vi "Send Cyclic to gRPC.vi"(8 "error in (no error)":errorcluster, 11 "CIFTemplatePlugin in":refnum<class "TemplatePlugin.lvclass">) -> (0 "error out":errorcluster, 3 "CIFTemplatePlugin out":refnum<class "TemplatePlugin.lvclass">)   [LabVIEW 2021, in "TemplatePlugin.lvclass"]
uses:
  TemplatePlugin.lvclass
  C:/Program Files/National Instruments/LabVIEW 2021/vi.lib/CIF Foundation/CIF Core/CIFCore/Class/CIFCorePlugin.lvclass
  <vilib>/CIF Foundation/CIF Core/CIFCore/Class/CIFCorePlugin.lvclass/CIFCorePlugin.ctl
  TemplatePlugin.lvclass/TemplatePlugin.ctl
  0c0f428d-7269-422d-ba27-f9d6fa7232ec.vi
  <vilib>/CIF Foundation/CIF CIPC/SubVIs/Check Error.vi
  <vilib>/CIF Foundation/CIF CIPC/SubVIs/Notify Of New Write.vi
  <vilib>/CIF Foundation/CIF CIPC/SubVIs/Get dll Path.vi
  <vilib>/CIF Foundation/CIF CIPC/SubVIs/Get Element Write Position.vi
  <vilib>/CIF Foundation/CIF CIPC/SubVIs/Get Element Info Variant.vi
  <vilib>/Utility/error.llb/Trim Whitespace.vi
  <vilib>/Utility/error.llb/Error Cluster From Error Code.vi
  <vilib>/CIF Foundation/CIF Core/CIFCore/Class/CIFCorePlugin.lvclass
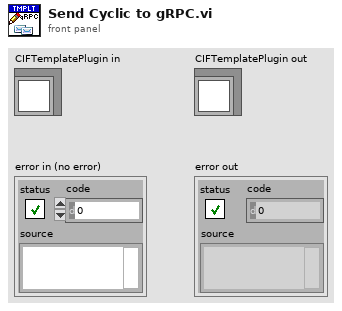
[diagram p1: front panel]
types:
  T1 = typedef "TemplateCommon.lvlib/To gRPC Cyclic Data.ctl" = cluster{"Data 1 -> gRPC":i32}
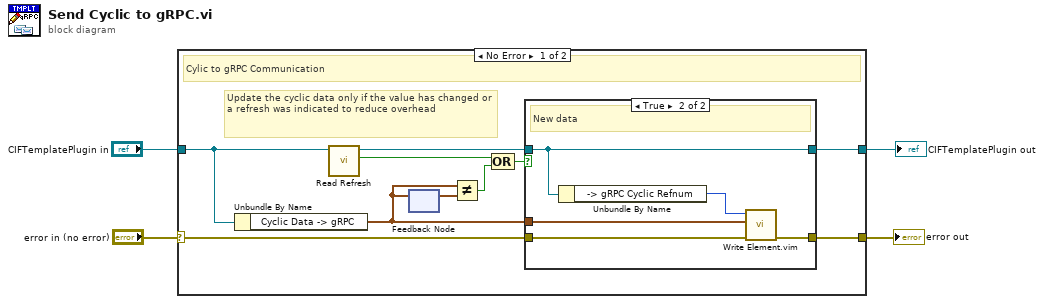
[diagram p0: block diagram]
diagram:
  n1 = case shown="No Error" "error in (no error)" {
    selector: "error in (no error)" -> [w10 w23]
    tunnel: [w11 w23] -> w3
    tunnel: [w12 w22] -> w1
    tunnel: "CIFTemplatePlugin in" -> [w9 w22]
    frame No Error {
      # "Update the cyclic data only if the value has changed or a refresh was indicated to reduce overhead"
      # "Cylic to gRPC Communication"
      n2 = Unbundle By Name(w9) -> ("Cyclic Data -> gRPC"=w13:T1)
      n3 = call <vilib>:"Read Refresh.vi"("CIFCorePlugin in"=w9) -> ("Refresh"=w6:bool, "CIFCorePlugin out"=w8:refnum<class "TemplatePlugin.lvclass">)  [unwired: 8 in, 1 out]
      n4 = feedback-in #1(w13) -> ()
      n5 = feedback #1() -> (w14:T1)  [unwired: 1 in]
      n6 = Not Equal?(x=w13, y=w14) -> (x != y?=w7:bool)
      n7 = Compound Arithmetic op=OR(w6, w7) -> (w5:bool)
      n8 = case shown="True" w5 {
        tunnel: w8 -> [w16 w21]
        tunnel: w13 -> [_ w19]
        tunnel: [w16 w21] -> w12
        tunnel: [w15 w17] -> w11
        tunnel: w10 -> [w15 w18]
        frame False {
        }
        frame True {
          # "New data"
          n9 = Unbundle By Name(w21) -> ("-> gRPC Cyclic Refnum"=w20:u64)
          n10 = call "Write Element.vim"("error in (no error)"=w18, "Data in"=w19, "CIPC Reference in"=w20) -> ("error out"=w17:errorcluster)  [unwired: 5 in, 3 out]
        }
      }
    }
    frame Error {
    }
  }
  "error out" <- w3
  "CIFTemplatePlugin out" <- w1
